vi "SetGetClass.vi"(7 "Set (f)":bool, 11 "Analysis In":refnum<class "AnalysisPluginsBase.lvclass">) -> (3 "Analysis Out":refnum<class "AnalysisPluginsBase.lvclass">)   [LabVIEW 2014, in "AnalysisPlugins.lvlib" / "AnalysisPluginsBase.lvclass"]
uses:
  AnalysisPluginsBase.lvclass
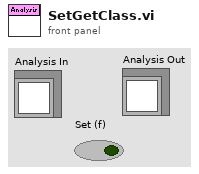
[diagram p1: front panel]
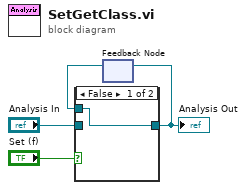
[diagram p0: block diagram]
diagram:
  n1 = feedback #1() -> (w1:refnum<class "AnalysisPluginsBase.lvclass">)  [unwired: 1 in]
  n2 = case shown="False" "Set (f)" {
    tunnel: [w5 w6] -> w2
    tunnel: "Analysis In" -> [_ w6]
    tunnel: w1 -> [w5 _]
    frame False {
    }
    frame True {
    }
  }
  "Analysis Out" <- w2
  n3 = feedback-in #1(w2) -> ()
